vi "jihoon.vi"() -> ()   [LabVIEW 2024]
panel:
  out "gap_flags.right":bool
  out "gap_flags.left":bool
  out "had_gaps":bool
  out "detected":bool
  out "timestamp":dbl
  out "valid":bool
  out "lane_departure_warning":bool
  out "right_curvature":dbl
  out "left_curvature":dbl
  out "center_offset":dbl
  in  "stop":bool
  out "steering_angle":dbl
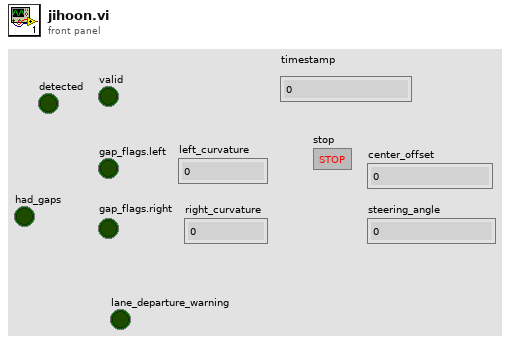
[diagram p1: front panel]
types:
  T1 = cluster{"timestamp":dbl, "path":cluster{"steering_angle":dbl, "center_offset":dbl, "left_curvature":dbl, "right_curvature":dbl, "lane_departure_warning":bool, "valid":bool}, "lane":cluster{"detected":bool, "had_gaps":bool, "gap_flags":cluster{"left":bool, "right":bool}}}
  T2 = cluster{"steering_angle":dbl, "center_offset":dbl, "left_curvature":dbl, "right_curvature":dbl, "lane_departure_warning":bool, "valid":bool}
  T3 = cluster{"detected":bool, "had_gaps":bool, "gap_flags":cluster{"left":bool, "right":bool}}
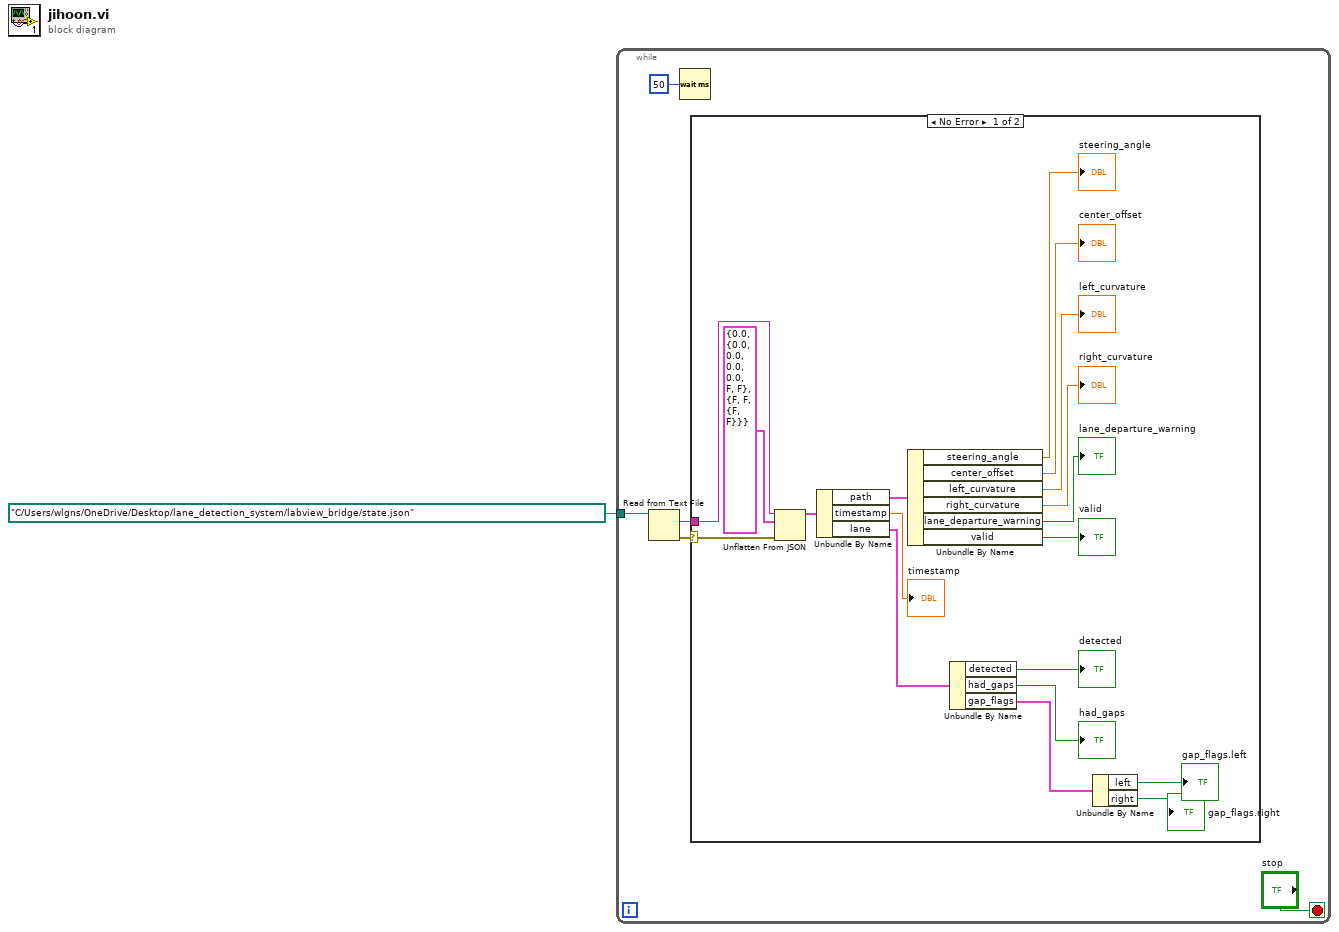
[diagram p0: block diagram]
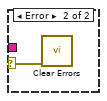
[diagram p2: hidden frame]
diagram:
  n1 = while {
    tunnel: path "C:/Users/wlgns/OneDrive/Desktop/lane_detection_system/labview_bridge/state.json" -> [w3]
    stop <- "stop" stop-if-true
    n2 = Read from Text File(file (use dialog)=w3) -> (text=w5:string, error out=w4:errorcluster)  [unwired: 3 in, 2 out]
    n3 = Wait (ms)(milliseconds to wait=u32 50 ("millisecond timer value")) -> ()  [unwired: 1 out]
    n4 = case shown="No Error" w4 {
      selector: w4 -> [w24 w25]
      tunnel: w5 -> [w23 _]
      frame No Error {
        n5 = Unflatten From JSON(JSON string=w23, type and defaults=T1 {"timestamp"=0.0, "path"={"steering_angle"=0.0, "center_offset"=0.0, "left_curvature"=0.0, "right_curvature"=0.0, "lane_departure_warning"=FALSE, "valid"=FALSE}, "lane"={"detected"=FALSE, "had_gaps"=FALSE, "gap_flags"={"left"=FALSE, "right"=FALSE}}} ("Cluster"), error in (no error)=w24) -> (value=w21:T1)  [unwired: 4 in, 1 out]
        n6 = Unbundle By Name(w21) -> ("path"=w20:T2, "timestamp"=→"timestamp":dbl, "lane"=w12:T3)
        n7 = Unbundle By Name(w20) -> ("steering_angle"=→"steering_angle":dbl, "center_offset"=→"center_offset":dbl, "left_curvature"=→"left_curvature":dbl, "right_curvature"=→"right_curvature":dbl, "lane_departure_warning"=→"lane_departure_warning":bool, "valid"=→"valid":bool)
        n8 = Unbundle By Name(w12) -> ("detected"=→"detected":bool, "had_gaps"=→"had_gaps":bool, "gap_flags"=w9:cluster{"left":bool, "right":bool})
        n9 = Unbundle By Name(w9) -> ("left"=→"gap_flags.left":bool, "right"=→"gap_flags.right":bool)
      }
      frame Error {
        n10 = call <vilib>:"Clear Errors.vi"("error in (no error)"=w25) -> ()  [unwired: 5 in, 2 out]
      }
    }
  }
